vi "pathPlanningOffensive.vi"(8 "error in (no error)":errorcluster, 10 "Line?":bool=TRUE, 11 "Game in":refnum<class "Game.lvclass">) -> (0 "error out":errorcluster, 3 "Game out":refnum<class "Game.lvclass">)   [LabVIEW 2020, in "Game.lvclass"]
uses:
  Game.lvclass
  Team_class/KeeperPlay.ctl
  Game.lvclass/Game.ctl
  Team_class/Team.lvclass/Team.ctl
  Read KeeperTeam.vi
  Team_class/Read KeeperPlay.vi
  Read OffensiveTeam.vi
  Team_class/Read RobotRef.vi
  Team_class/Write RobotRef.vi
  Write RRTTeam.vi
  Ally_class/Ally.lvclass
  C:/RoboIME/SSL_AI/Team_class/Team.lvclass
  Robot_class/Robot.lvclass
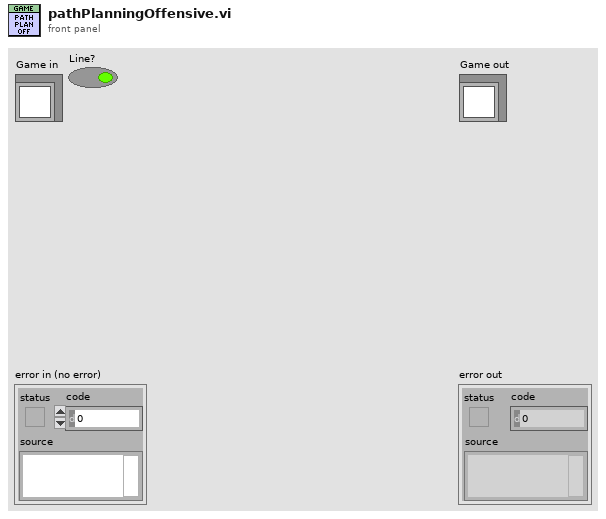
[diagram p1: front panel]
types:
  T1 = typedef "KeeperPlay.ctl" = enum16{"ZigZag", "BallPlacement", "Goto", "NormalGame", "KeeperPlay", "Halt", "Timeout", "PenaltyEnemy", "TestPlay"}
  T2 = typedef "AI Input.ctl" = cluster{"our_robots":T3[], "enemy_robots":T3[], "balls":T11[], "geometry":T12, "IA Judge":T13, "Received Timestamp":timestamp, "Events":T15}
  T3 = typedef "AI Robot.ctl" = cluster{"id":u32, "function":T4, "x":dbl, "y":dbl, "orientation":dbl, "v_tangent":dbl, "v_normal":dbl, "v_ang":dbl, "kick_x":dbl, "kick_z":dbl, "dribble":bool, "Timestamp":timestamp, "estimatives":T5, "dest_x_kick":dbl, "dest_y_kick":dbl, "Gap Coord":dbl[], "States":T6, "Path ":dbl[][], "Path  Smooth":dbl[][], "Dest":T7, "vx_desired":dbl, "vy_desired":dbl, "slowBehavior":bool, "VSSStates":T9, "robotKickState":T10}
  T4 = typedef "Functions Enum.ctl" = enum16{"2nd Striker", "Attacker", "Goalie", "Defender", "Striker", "Goto 0", "Dummy", "Kicker", "ZigZag 0", "ZigZag 1", "ZigZag 2", "ZigZag 3", "ZigZag 4", "ZigZag 5", "ZigZag 6", "ZigZag 7", "ZigZag 8", ""}
  T5 = typedef "estimatives.ctl" = cluster{"est_v_tangent":dbl, "est_v_normal":dbl, "est_vx":dbl, "est_vy":dbl, "Pos Robot Est":dbl[], "est_v_ang":dbl}
  T6 = typedef "AttackerStates.ctl" = enum16{"Pass", "GoToTangent", "BallGetting", "GoToKick", ""}
  T7 = typedef "PathDests.ctl" = T8[]
  T8 = typedef "PathDest.ctl" = cluster{"dest_x":dbl, "dest_y":dbl, "dest_orientation":dbl, "dest_vel":dbl}
  T9 = typedef "VSSAttackerStates.ctl" = enum16{"Pass", "GoToTangent", "BallGetting", "GoToKick", "Rotate anti-clockwise", "Rotate Clockwise", ""}
  T10 = typedef "robotKickToStates.ctl" = enum16{"avoidCollideBall", "goToBackBall", "none", "andar", "girar", "chutar"}
  T11 = typedef "AI Ball.ctl" = cluster{"x":dbl, "y":dbl, "timestamp":timestamp, "Vel_x":dbl, "Vel_y":dbl, "Pos Bola Est":dbl[], "Valid":bool, "z":dbl, "Vel_z":dbl}
  T12 = typedef "Field Size.ctl" = cluster{"line_width":u32, "field_length":u32, "field_width":u32, "boundary_width":u32, "referee_width":u32, "goal_width":u32, "goal_depth":u32, "goal_wall_width":u32, "center_circle_radius":u32, "defense_radius":u32, "defense_stretch":u32, "free_kick_from_defense_dist":u32, "penalty_spot_from_field_line_dist":u32, "penalty_line_from_spot_dist":u32}
  T13 = typedef "AI Judge.ctl" = cluster{"stage":string, "command":string, "our_goalie_id":dbl, "enemy_goalie_id":dbl, "command enum":T14, "Time":enum16{"Azul", "Amarelo"}, "Point":cluster{"x":sgl, "y":sgl}}
  T14 = typedef "Command Enum.ctl" = enum16{"Halt", "Stop", "Force Start", "PKA Normal Start", "Prepare Kickoff Ally", "PKE Normal Start", "Prepare Kickoff Enemy", "Prepare Penalty Ally", "PPA Normal Start", "Prepare Penalty Enemy", "PPE Normal Start", "Direct Free Enemy", "Direct Free Ally", "Indirect Free Enemy", "Indirect Free Ally", "Timeout Enemy", "Timeout Ally", "Goal Enemy", "Goal Ally", "Ball Placement Enemy", "Ball Placement Ally", "Normal Half Time", "Extra Time Break", "Extra Half Time", "None", "Post Game"}
  T15 = typedef "Events.ctl" = cluster{"Touch":bool, "Ball out":bool, "id touch":dbl, "Ball out of \nVision":bool, "Ball inside \nGoalie area":bool, "Robot not responding":bool, "Robots responding status":dbl[], "Enemy Ball \nPossession":bool, "Pass State":bool, "id end of pass":dbl, "Kick":bool, "Id ini Possession":dbl, "Ball Possesion":bool, "Id Possesion":dbl, "Direct Kick":bool, "2nd Strk Ativo":bool}
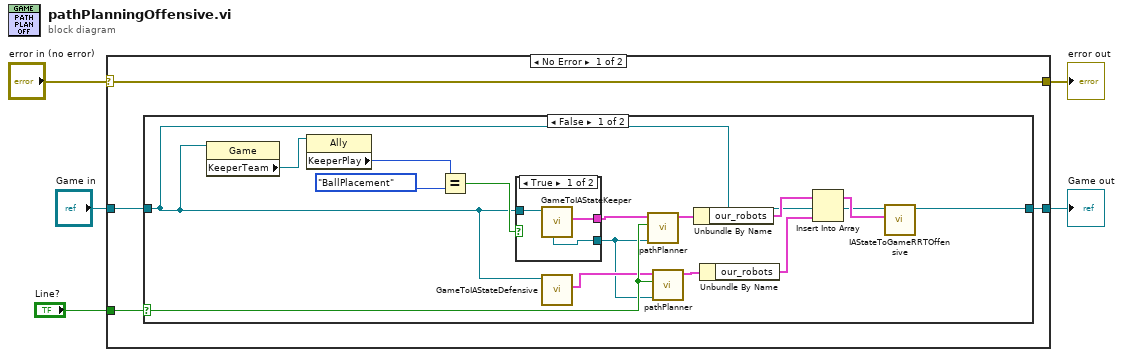
[diagram p0: block diagram]
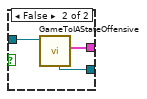
[diagram p2: hidden frame]
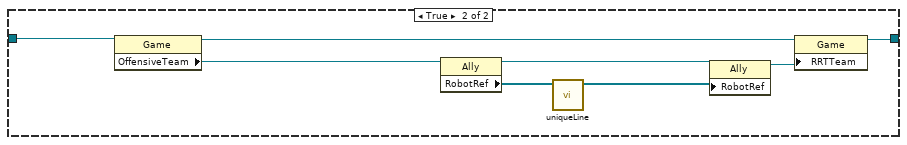
[diagram p3: hidden frame]
diagram:
  n1 = case shown="No Error" "error in (no error)" {
    selector: "error in (no error)" -> [w9 w40]
    tunnel: [w9 w40] -> w4
    tunnel: [w7 w39] -> w2
    tunnel: "Game in" -> [w8 w39]
    tunnel: "Line?" -> [w6 _]
    frame No Error {
      n2 = case shown="False" w6 {
        selector: w6 -> [w15 _]
        tunnel: w8 -> [w12 w38]
        tunnel: [w22 w31] -> w7
        frame False {
          n3 = property class="Game"(reference=w12) -> ("KeeperTeam"=w21:refnum<class "Ally.lvclass">)  [unwired: 1 in, 2 out]
          n4 = property class="Ally"(reference=w21) -> ("KeeperPlay"=w20:T1)  [unwired: 1 in, 2 out]
          n5 = Equal?(x=w20, y=KeeperPlay."BallPlacement" ("KeeperPlay")) -> (x = y?=w18:bool)
          n6 = case shown="True" w18 {
            tunnel: [w26 w30] -> w23
            tunnel: [w25 w29] -> w10
            tunnel: w12 -> [w27 w28]
            frame True {
              n7 = call-dynamic "GameToIAStateKeeper.vi"("Game in"=w27) -> ("IA State out"=w26:T2, "Parameters.lvclass"=w25:refnum<class "Parameters.lvclass">)  [unwired: 7 in, 2 out]
            }
            frame False {
              n8 = call-dynamic "GameToIAStateOffensive.vi"("Game in"=w28) -> ("IA State out"=w30:T2, "Parameters.lvclass"=w29:refnum<class "Parameters.lvclass">)  [unwired: 6 in, 3 out]
            }
          }
          n9 = call "GameToIAStateDefensive.vi"("Game in"=w12) -> ("IA State out"=w11:T2)  [unwired: 8 in, 2 out]
          n10 = call "pathPlanner.vi"("Parameters.lvclass"=w10, "Line?"=w15, "IA State Output in"=w23) -> ("IA State Output out"=w24:T2)  [unwired: 8 in]
          n11 = call "pathPlanner.vi"("Parameters.lvclass"=w10, "Line?"=w15, "IA State Output in"=w11) -> ("IA State Output out"=w14:T2)  [unwired: 8 in]
          n12 = Unbundle By Name(w24) -> ("our_robots"=w17:T3[])
          n13 = Unbundle By Name(w14) -> ("our_robots"=w13:T3[])
          n14 = Insert Into Array(array=w17, new element=w13) -> (w16:T3[])  [unwired: 1 in]
          n15 = call-dynamic "IAStateToGameRRTOffensive.vi"("our_robots"=w16, "Game in"=w12) -> ("Game out"=w22:refnum<class "Game.lvclass">)  [unwired: 8 in, 1 out]
        }
        frame True {
          n16 = property class="Game"(reference=w38) -> (reference out=w33:refnum<class "Game.lvclass">, "OffensiveTeam"=w37:refnum<class "Ally.lvclass">)  [unwired: 1 in, 1 out]
          n17 = property class="Ally"(reference=w37) -> (reference out=w34:refnum<class "Ally.lvclass">, "RobotRef"=w36:refnum<class "Robot.lvclass">[])  [unwired: 1 in, 1 out]
          n18 = call "uniqueLine.vi"("RobotRef in"=w36) -> ("RoboRef out"=w35:refnum<class "Robot.lvclass">[])  [unwired: 10 in]
          n19 = property class="Ally"(reference=w34, "RobotRef"=w35) -> (reference out=w32:refnum<class "Ally.lvclass">)  [unwired: 1 in, 1 out]
          n20 = property class="Game"(reference=w33, "RRTTeam"=w32) -> (reference out=w31:refnum<class "Game.lvclass">)  [unwired: 1 in, 1 out]
        }
      }
    }
    frame Error {
    }
  }
  "error out" <- w4
  "Game out" <- w2
